vi "Update Status.vi"(8 "error in (no error)":errorcluster caption="entrée d'erreur (pas d'erreur)", 10 "DAQmx Tasks":T1(array[cluster]), 11 "DAQmxTaskContainer en entrée":refnum<class "DAQmxTaskContainer.lvclass">) -> (0 "error out":errorcluster caption="sortie d'erreur", 2 "DAQmx Tasks out":T1(array[cluster]), 3 "DAQmxTaskContainer en sortie":refnum<class "DAQmxTaskContainer.lvclass">)   [LabVIEW 2015, in "DAQmxTaskContainer.lvclass"]
uses:
  DAQmxTaskContainer/DAQmxTaskContainer.lvclass
  DAQmxTaksContainer_General.lvclass
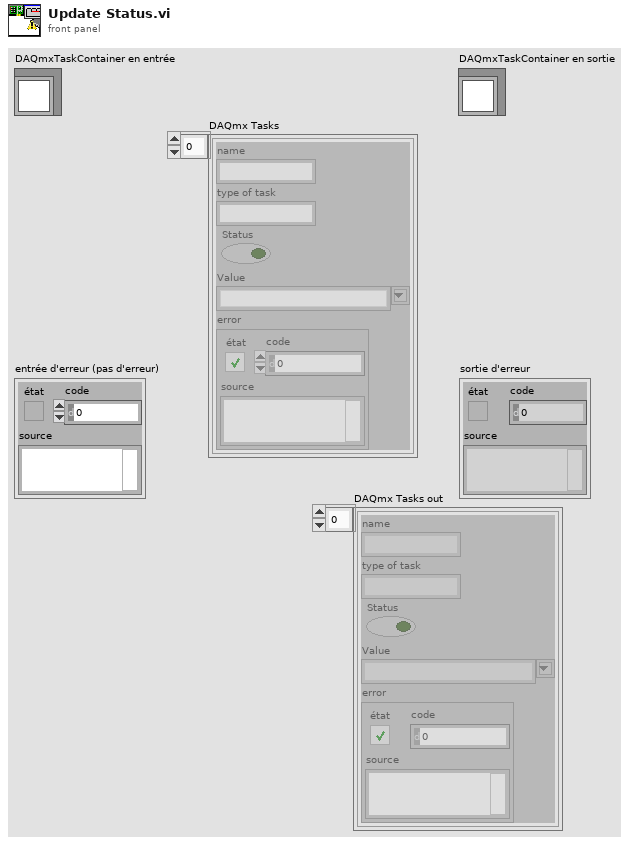
[diagram p1: front panel]
types:
  T1 = cluster{"name":string, "type of task":string, "Status":bool, "Value":string, "error":errorcluster}[]
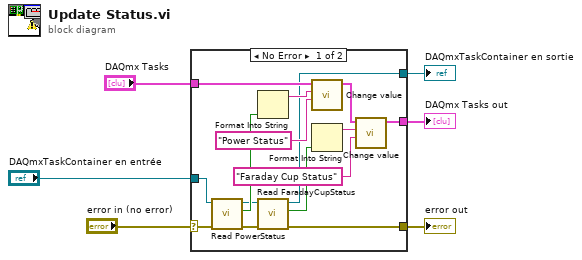
[diagram p0: block diagram]
diagram:
  n1 = case shown="No Error" "error in (no error)" {
    selector: "error in (no error)" -> [w7 w24]
    tunnel: [w11 w24] -> w5
    tunnel: [w8 w23] -> w3
    tunnel: "DAQmxTaskContainer en entrée" -> [w9 w23]
    tunnel: "DAQmx Tasks" -> [w21 w22]
    tunnel: [w15 w22] -> w1
    frame No Error {
      n2 = call "Read PowerStatus.vi"("error in (no error)"=w7, "DAQmxTaksContainer_General in"=w9) -> ("error out"=w12:errorcluster, "PowerStatus"=w13:bool, "DAQmxTaksContainer_General out"=w10:refnum<class "DAQmxTaskContainer.lvclass">)  [unwired: 7 in]
      n3 = Format Into String(w13) -> (resulting string=w20:string)  [unwired: 3 in, 1 out]
      n4 = call "Read FaradayCupStatus.vi"("error in (no error)"=w12, "DAQmxTaksContainer_General in"=w10) -> ("error out"=w11:errorcluster, "FaradayCupStatus"=w14:bool, "DAQmxTaksContainer_General out"=w8:refnum<class "DAQmxTaskContainer.lvclass">)  [unwired: 7 in]
      n5 = call "Change value.vi"("Task name"="Power Status", "Data string"=w20, "DAQmx Tasks"=w21) -> ("tableau en sortie"=w17:T1)  [unwired: 8 in]
      n6 = Format Into String(w14) -> (resulting string=w18:string)  [unwired: 3 in, 1 out]
      n7 = call "Change value.vi"("Task name"="Faraday Cup Status", "Data string"=w18, "DAQmx Tasks"=w17) -> ("tableau en sortie"=w15:T1)  [unwired: 8 in]
    }
    frame Error {
    }
  }
  "error out" <- w5
  "DAQmxTaskContainer en sortie" <- w3
  "DAQmx Tasks out" <- w1
